vi "Image Processing Handler Create.vi"(5 "Camera? (F)":bool, 6 "data queue":refnum<queue>, 7 "Video Processor":refnum<class "Video Processor.lvclass">, 8 "error in (no error)":errorcluster, 10 "Image Ctl Refnum":refnum<vi>, 11 "Image Processing Handler in":refnum<class "Image Processing Handler.lvclass">) -> (0 "error out":errorcluster, 3 "Image Processing Handler out":refnum<class "Image Processing Handler.lvclass">)   [LabVIEW 2018, in "Image Processing Handler.lvclass"]
uses:
  Image Processing Handler.lvclass
  Message/Message.lvclass
  Video Processor/Video Processor.lvclass
  Image Processing Handler.lvclass/Image Processing Handler.ctl
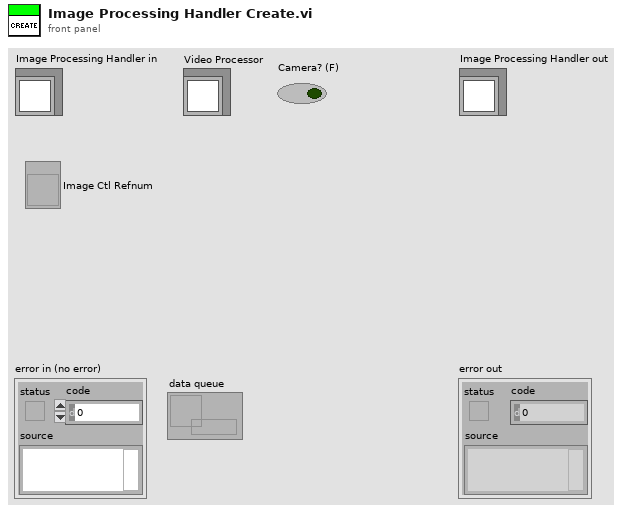
[diagram p1: front panel]
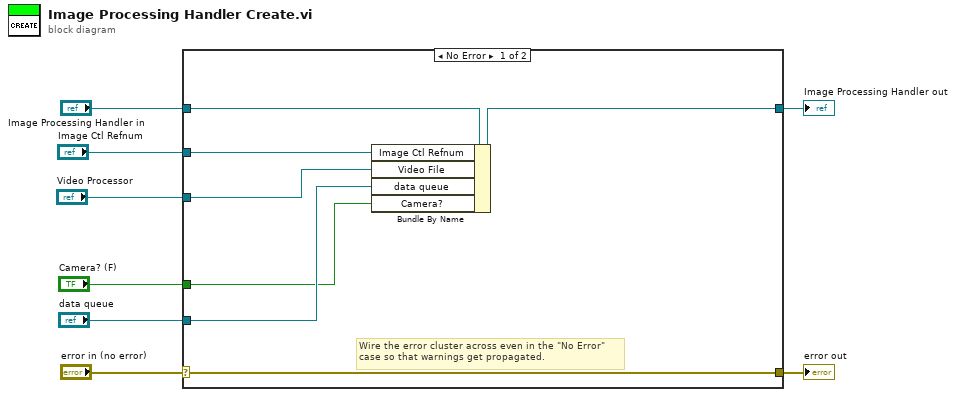
[diagram p0: block diagram]
diagram:
  n1 = case shown="No Error" "error in (no error)" {
    selector: "error in (no error)" -> [w15 w17]
    tunnel: [w15 w17] -> w7
    tunnel: [w13 w16] -> w5
    tunnel: "Image Processing Handler in" -> [w14 w16]
    tunnel: "data queue" -> [w11 _]
    tunnel: "Image Ctl Refnum" -> [w12 _]
    tunnel: "Video Processor" -> [w10 _]
    tunnel: "Camera? (F)" -> [w9 _]
    frame No Error {
      # "Wire the error cluster across even in the \"No Error\"\ncase so that warnings get propagated."
      n2 = Bundle By Name(cluster=w14, "Image Ctl Refnum"=w12, "Video File"=w10, "data queue"=w11, "Camera?"=w9) -> (w13:refnum<class "Image Processing Handler.lvclass">)
    }
    frame Error {
    }
  }
  "error out" <- w7
  "Image Processing Handler out" <- w5
